vi "Start Point.vi"(5 "Series Enqueuer":refnum<class "Message Enqueuer.lvclass">, 7 "Point Ident":string, 8 "error in":errorcluster, 11 "MSS in":refnum<class "Measure and Stimulus Subsystems.lvclass">) -> (0 "error out":errorcluster, 3 "MSS out":refnum<class "Measure and Stimulus Subsystems.lvclass">)   [LabVIEW 2023, in "HAL GOOP4.lvlib" / "Measure and Stimulus Subsystems.lvclass"]
uses:
  Measure and Stimulus Subsystems.lvclass
  <vilib>/ActorFramework/Message Enqueuer/Message Enqueuer.lvclass
  Measure and Stimulus Subsystems.lvclass/Measure and Stimulus Subsystems.ctl
  Virt Instr Host/Virt Instr Local.lvclass
  Series/ISeries Actor/ISeries Actor Messages/Start Point on Target Msg/Start Point on Target Msg.lvclass
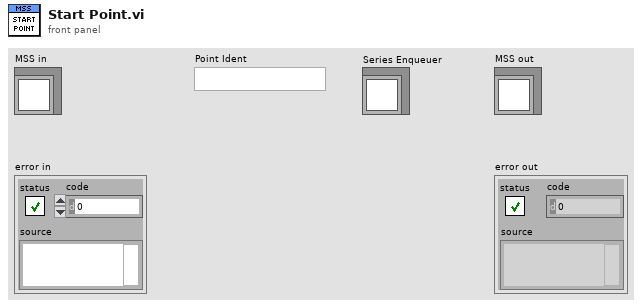
[diagram p1: front panel]
types:
  T1 = map{string, refnum<class "Virt Instr Local.lvclass">}
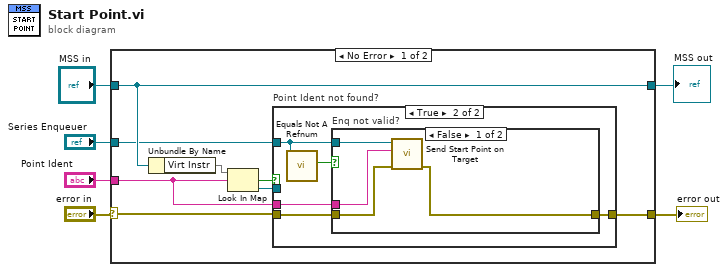
[diagram p0: block diagram]
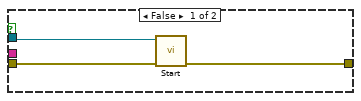
[diagram p2: hidden frame]
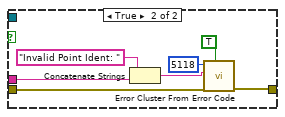
[diagram p3: hidden frame]
diagram:
  n1 = case shown="No Error" "error in" {
    selector: "error in" -> [w10 w35]
    tunnel: [w14 w35] -> w6
    tunnel: "MSS in" -> [w9 w34]
    tunnel: "Point Ident" -> [w8 _]
    tunnel: [w9 w34] -> w2
    tunnel: "Series Enqueuer" -> [w7 _]
    frame No Error {
      n2 = Unbundle By Name(w9) -> ("Virt Instr"=w13:T1)
      n3 = Look In Map(map=w13, key=w8) -> (key not found?=w11:bool, value=w12:refnum<class "Virt Instr Local.lvclass">)  [unwired: 1 in]
      n4 = case "Point Ident not found?" shown="True" w11 {
        tunnel: w12 -> [w16 _]
        tunnel: w10 -> [w17 w21]
        tunnel: [w15 w22] -> w14
        tunnel: w8 -> [_ w20]
        tunnel: w7 -> [_ w18]
        frame False {
          n5 = call-dynamic "Start.vi"("error in (no error)"=w17, "Virt Instr Base in"=w16) -> ("error out"=w15:errorcluster)  [unwired: 8 in, 1 out]
        }
        frame True {
          n6 = call <vilib>:"Equals Not A Refnum.vi"("Message Enqueuer"=w18) -> ("Not a refnum?"=w19:bool)  [unwired: 10 in]
          n7 = case "Enq not valid?" shown="False" w19 {
            tunnel: [w23 w27] -> w22
            tunnel: w21 -> [w25 w28]
            tunnel: w20 -> [w24 w30]
            tunnel: w18 -> [w26 _]
            frame False {
              n8 = call "Send Start Point on Target.vi"("error in (no error)"=w25, "Point Ident"=w24, "Message Enqueuer"=w26) -> ("error out"=w23:errorcluster)  [unwired: 7 in, 1 out]
            }
            frame True {
              n9 = Concatenate Strings("Invalid Point Ident: ", w30) -> (w31:string)
              n10 = call <vilib>:"Error Cluster From Error Code.vi"("show call chain? (False)"=TRUE, "error in (no error)"=w28, "error message (\"\")"=w31, "error code (0)"=5118) -> ("error out"=w27:errorcluster)  [unwired: 5 in]
            }
          }
        }
      }
    }
    frame Error {
    }
  }
  "error out" <- w6
  "MSS out" <- w2
